vi "MenuActive(Root).vi"(8 "error in (no error)":errorcluster caption="错误输入（无错误）", 10 "菜单引用":refnum<k9>, 11 "PanelDataNode 输入":refnum<class "PanelDataNode.lvclass"> caption="DNL_LabVIEW Object in") -> (0 "error out":errorcluster caption="错误输出", 3 "PanelDataNode 输出":refnum<class "PanelDataNode.lvclass"> caption="DNL_LabVIEW Object out")   [LabVIEW 2016, in "PanelRootNode.lvclass"]
uses:
  PanelRootNode.lvclass
  PanelDataNode/PanelDataNode.lvclass
  PanelDataNode/PanelDataNode.lvclass/PanelDataNode.ctl
panel:
  out "menu reference out":refnum<k9>
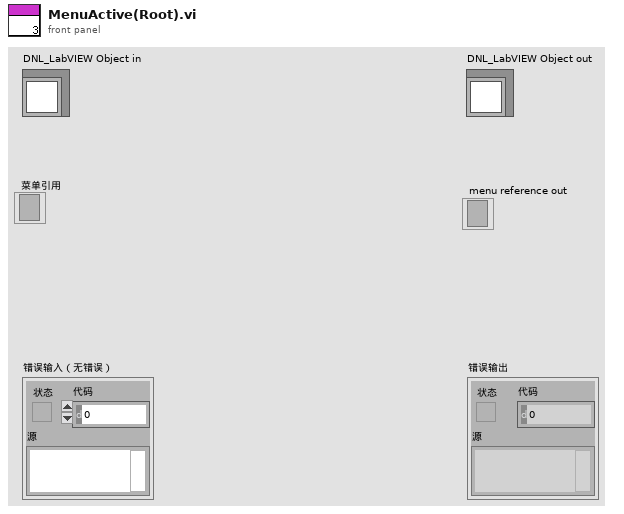
[diagram p1: front panel]
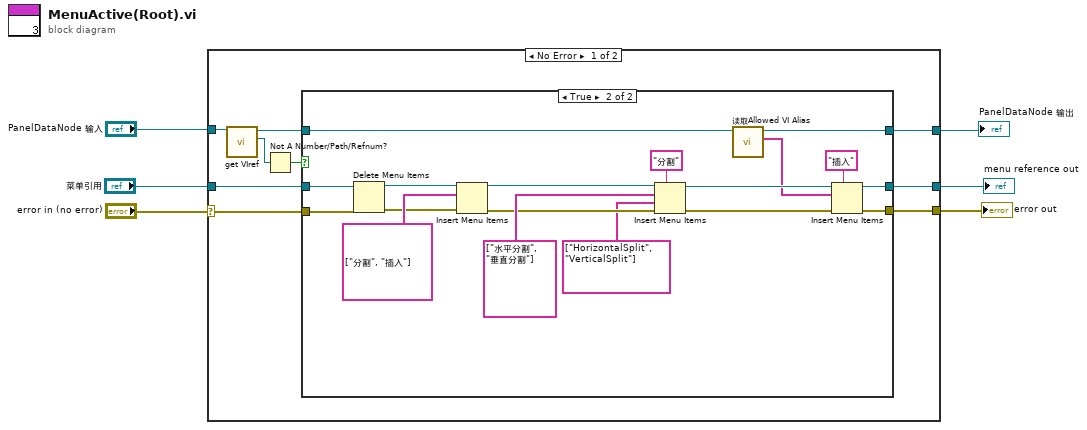
[diagram p0: block diagram]
diagram:
  n1 = case shown="No Error" "error in (no error)" {
    selector: "error in (no error)" -> [w13 w39]
    tunnel: [w14 w38] -> w5
    tunnel: [w15 w39] -> w4
    tunnel: "PanelDataNode 输入" -> [w9 w38]
    tunnel: "菜单引用" -> [w8 w37]
    tunnel: [w7 w37] -> w1
    frame No Error {
      n2 = call "get VIref.vi"("PanelDataNode输入"=w9) -> ("VI*"=w11:refnum<vi>, "PanelDataNode输出"=w12:refnum<class "PanelDataNode.lvclass">)  [unwired: 8 in, 1 out]
      n3 = Not A Number/Path/Refnum?(number/path/refnum=w11) -> (NaN/Path/Refnum?=w10:bool)
      n4 = case shown="True" w10 {
        tunnel: [w17 w27] -> w15
        tunnel: w12 -> [w18 w25]
        tunnel: [w18 w23] -> w14
        tunnel: w13 -> [w17 w21]
        tunnel: w8 -> [w16 w20]
        tunnel: [w16 w19] -> w7
        frame False {
        }
        frame True {
          n5 = Delete Menu Items(6:w21, 9:w20) -> (0:w31:errorcluster, 3:w36:refnum<k9>)  [unwired: 2 in]
          n6 = Insert Menu Items(6:w31, 8:string[] ["分割", "插入"] ("项名称"), 9:w36) -> (0:w30:errorcluster, 3:w34:refnum<k9>)  [unwired: 3 in, 1 out]
          n7 = Insert Menu Items(5:"分割" ("菜单标识符"), 6:w30, 7:string[] ["HorizontalSplit", "VerticalSplit"] ("项标识符"), 8:string[] ["水平分割", "垂直分割"] ("项名称"), 9:w34) -> (0:w22:errorcluster, 3:w28:refnum<k9>)  [unwired: 1 in, 1 out]
          n8 = call "读取Allowed VI Alias.vi"("PanelDataNode输入"=w25) -> ("Allowed VI Alias"=w24:string[], "PanelDataNode输出"=w23:refnum<class "PanelDataNode.lvclass">)  [unwired: 8 in, 1 out]
          n9 = Insert Menu Items(5:"插入" ("菜单标识符"), 6:w22, 8:w24, 9:w28) -> (0:w27:errorcluster, 3:w19:refnum<k9>)  [unwired: 2 in, 1 out]
        }
      }
    }
    frame Error {
    }
  }
  "error out" <- w4
  "PanelDataNode 输出" <- w5
  "menu reference out" <- w1
